vi "Capture single frame.vi"(7 "Error In":errorcluster, 8 "Gain in":i32 min=0 max=2000 step=1, 9 "Exposure time (ms)":dbl, 10 "Camera reference in":refnum<k24>) -> (0 "Error Out":errorcluster, 2 "Array":u16[][](array[numeric]), 3 "Camera reference out":refnum<k24>)   [LabVIEW 2017]
uses:
  C:/Program Files/National Instruments/LabVIEW 2017/instr.lib/IDS/ueye.NET/uEyeDotNet.dll
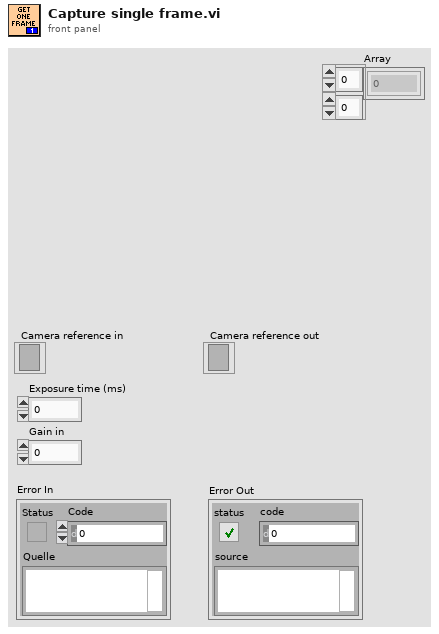
[diagram p1: front panel]
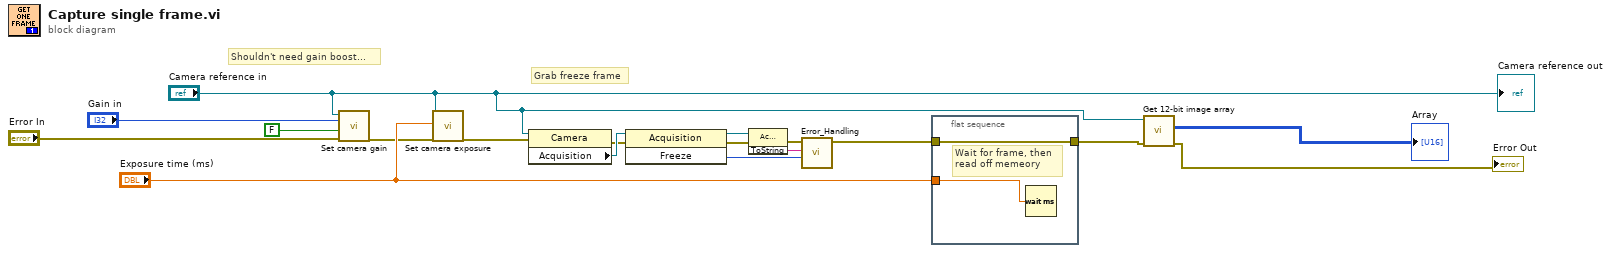
[diagram p0: block diagram]
diagram:
  # "Grab freeze frame"
  # "Shouldn't need gain boost..."
  n1 = call "Set camera gain.vi"("Error In"="Error In", "Gain Boost in"=FALSE, "Gain in"="Gain in", ".NET (Reference)"="Camera reference in") -> ("Error Out"=w4:errorcluster)  [unwired: 5 in, 2 out]
  n2 = call "Set camera exposure.vi"("Camera reference in"="Camera reference in", "Exposure time (ms)"="Exposure time (ms)", "Error In"=w4) -> ("Error Out"=w3:errorcluster)  [unwired: 15 in, 1 out]
  n3 = property class="Camera"(reference="Camera reference in", error in=w3) -> (error out=w15:errorcluster, "Acquisition"=w16:refnum<k24>)  [unwired: 1 out]
  n4 = invoke class="Acquisition" method="Freeze"(reference=w16, error in=w15) -> (reference out=w11:refnum<k24>, error out=w12:errorcluster, "Freeze"=w10:i32)  [unwired: 1 in]
  n5 = invoke class="Acquisition" method="ToString"(reference=w11, error in=w12) -> (error out=w14:errorcluster, "ToString"=w13:string)  [unwired: 1 in, 1 out]
  n6 = call <instrlib>:"Error_Handling.vi"("Error Code"=w10, "Error String"=w13, "Error In"=w14) -> ("Error Out"=w7:errorcluster)  [unwired: 8 in]
  n7 = flat-sequence {
    tunnel: w7 -> [w20]
    tunnel: [w20] -> w6
    tunnel: "Exposure time (ms)" -> [w19]
    frame #0 {
      # "Wait for frame, then\nread off memeory"
      n8 = Wait (ms)(milliseconds to wait=w19) -> ()  [unwired: 1 out]
    }
  }
  n9 = call "Get 12-bit image array.vi"("Error In"=w6, "Camera reference in"="Camera reference in") -> ("Error Out"=→"Error Out":errorcluster, "Array"=→"Array":u16[][])  [unwired: 6 in, 1 out]
  "Camera reference out" <- "Camera reference in"
